vi "MGCC_StaEst_initial_input_RTDS.vi"() -> (0 "error out":errorcluster)   [LabVIEW 2016]
uses:
  <vilib>/Utility/error.llb/Error Cluster From Error Code.vi
  <vilib>/ErrorRing/Error Ring.xnode
panel:
  out "element":i32
  out "size(s)":i32[](array[numeric])
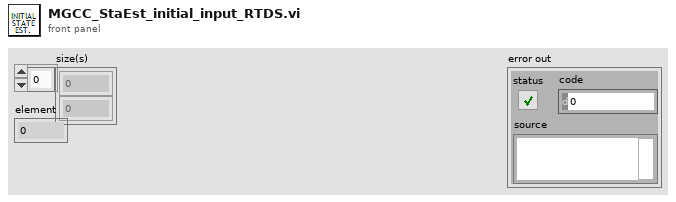
[diagram p1: front panel]
types:
  T1 = cluster{"V_node":cdb[][], "P_node":cdb[][], "I_node":cdb[][], "NumN":dbl, "NumL":dbl, "Ybus":cdb[][], "sspn":dbl[][], "ssqn":dbl[][], "ssvn":dbl[][], "SlackBus":dbl, "Topology":dbl[][]}
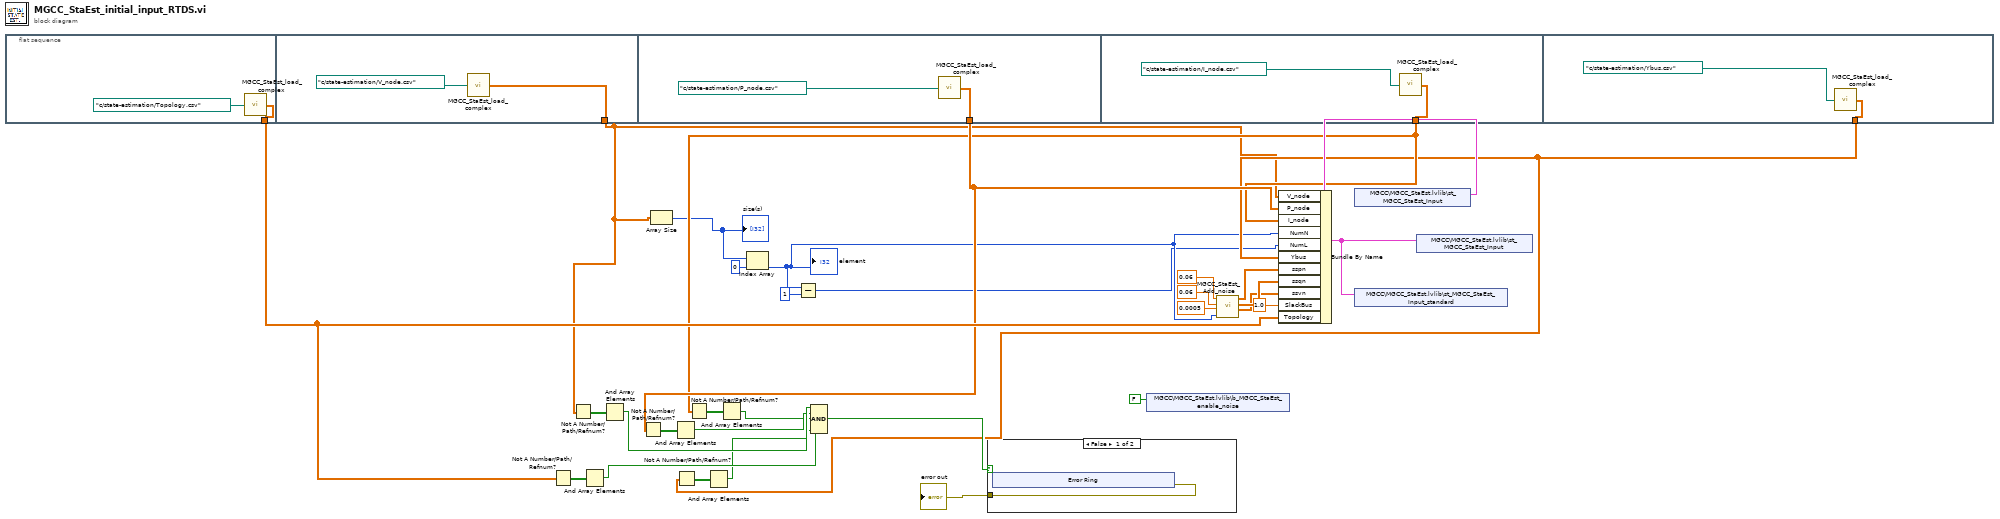
[diagram p0: block diagram]
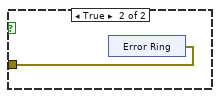
[diagram p2: hidden frame]
diagram:
  n1 = flat-sequence {
    tunnel: [w33] -> w13
    tunnel: [w35] -> w7
    tunnel: [w37] -> w12
    tunnel: [w39] -> w11
    tunnel: [w41] -> w9
    frame #0 {
      n2 = call "MGCC_StaEst_load_complex.vi"("file path (dialog if empty)"=path "c:/state-estimation/Topology.csv" ("file path (use dialog)")) -> ("Array 13"=w33:cdb[][])
    }
    frame #1 {
      n3 = call "MGCC_StaEst_load_complex.vi"("file path (dialog if empty)"=path "c:/state-estimation/V_node.csv" ("file path (use dialog)")) -> ("Array 13"=w35:cdb[][])
    }
    frame #2 {
      n4 = call "MGCC_StaEst_load_complex.vi"("file path (dialog if empty)"=path "c:/state-estimation/P_node.csv" ("file path (use dialog)")) -> ("Array 13"=w37:cdb[][])
    }
    frame #3 {
      n5 = call "MGCC_StaEst_load_complex.vi"("file path (dialog if empty)"=path "c:/state-estimation/I_node.csv" ("file path (use dialog)")) -> ("Array 13"=w39:cdb[][])
    }
    frame #4 {
      n6 = call "MGCC_StaEst_load_complex.vi"("file path (dialog if empty)"=path "c:/state-estimation/Ybus.csv" ("file path (use dialog)")) -> ("Array 13"=w41:cdb[][])
    }
  }
  n7 = Not A Number/Path/Refnum?(number/path/refnum=w13) -> (NaN/Path/Refnum?=w22:bool[][])
  n8 = Not A Number/Path/Refnum?(number/path/refnum=w7) -> (NaN/Path/Refnum?=w21:bool[][])
  n9 = And Array Elements(Boolean array=w22) -> (logical AND=w15:bool)
  n10 = And Array Elements(Boolean array=w21) -> (logical AND=w18:bool)
  n11 = Not A Number/Path/Refnum?(number/path/refnum=w12) -> (NaN/Path/Refnum?=w19:bool[][])
  n12 = Array Size(array=w7) -> (size(s)=w6:i32[])
  "size(s)" <- w6
  n13 = And Array Elements(Boolean array=w19) -> (logical AND=w17:bool)
  n14 = Not A Number/Path/Refnum?(number/path/refnum=w9) -> (NaN/Path/Refnum?=w10:bool[][])
  n15 = Not A Number/Path/Refnum?(number/path/refnum=w11) -> (NaN/Path/Refnum?=w20:bool[][])
  n16 = And Array Elements(Boolean array=w10) -> (logical AND=w8:bool)
  n17 = And Array Elements(Boolean array=w20) -> (logical AND=w16:bool)
  n18 = Index Array(array=w6, index=0) -> (element=w3:i32)
  "element" <- w3
  n19 = Subtract(x=w3, y=1) -> (x-y=w2:i32)
  n20 = Compound Arithmetic op=AND(w18, w17, w16, w15, w8) -> (w14:bool)
  n21 = case shown="False" w14 {
    tunnel: [w43 w49] -> w1
    frame False {
      n22 = xnode "Error Ring"() -> ("error out"=w43:errorcluster)
    }
    frame True {
      n23 = xnode "Error Ring"() -> ("error out"=w49:errorcluster)
    }
  }
  "error out" <- w1
  n24 = shared-variable "MGCC\\MGCC_StaEst.lvlib\\b_MGCC_StaEst_enable_noise"(FALSE ("b_MGCC_StaEst_enable_noise")) -> ()  [unwired: 1 in, 1 out]
  n25 = call "MGCC_StaEst_Add_noise.vi"("spn"=0.06, "sqn"=0.06, "svn"=0.0005, "Node"=w3) -> ("sspn"=w25:dbl[][], "ssvn"=w24:dbl[][], "ssqn"=w23:dbl[][])  [unwired: 2 in]
  n26 = shared-variable "MGCC\\MGCC_StaEst.lvlib\\st_MGCC_StaEst_Input"() -> (w30:T1)  [unwired: 1 in, 1 out]
  n27 = Bundle By Name(cluster=w30, "V_node"=w7, "P_node"=w12, "I_node"=w11, "NumN"=w3, "NumL"=w2, "Ybus"=w9, "sspn"=w25, "ssqn"=w24, "ssvn"=w23, "SlackBus"=1.0, "Topology"=w13) -> (w29:T1)
  n28 = shared-variable "MGCC\\MGCC_StaEst.lvlib\\st_MGCC_StaEst_Input_standard"(w29) -> ()  [unwired: 1 in, 1 out]
  n29 = shared-variable "MGCC\\MGCC_StaEst.lvlib\\st_MGCC_StaEst_Input"(w29) -> ()  [unwired: 1 in, 1 out]
